vi "Solver1.vi"(10 "Word List":string[](array[string]), 11 "Word Search Grid":string[][](array[string])) -> (3 "Solutions":T2)   [LabVIEW 2022 SP3]
uses:
  support/Solutions--map.ctl
  support/Letter Index--cluster.ctl
panel:
  out "Array":T1[](array[typedef])
  # "Implement your Word Search challenge solution in this VI. Do not change the connector pane of this VI."
  # "Letters will always be ALL CAPS."
  # "Words will always be ALL CAPS."
  # "The Word Search Grid contains the 2D array of letters in which all words in the Word List appear. Words can appear forwards, backwards, up, down, and diagonally in any direction.\n\nThe Solutions map will contain one entry per item in the Word List. The map elements are:\n\nWord: The word from the Word List.\nLetter Indices: The row/column indices into the Word Search Grid for each letter (in order) in the word."
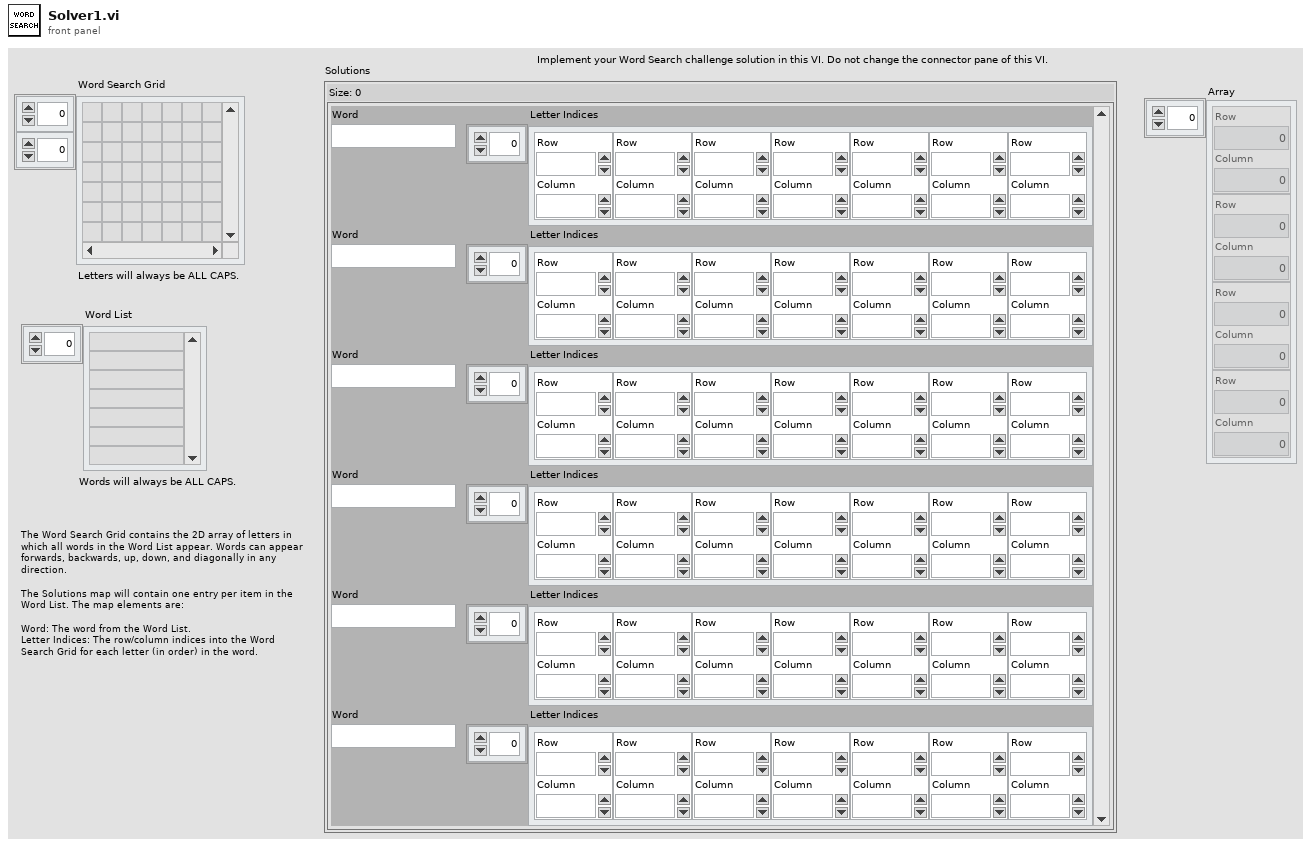
[diagram p1: front panel]
types:
  T1 = typedef "Letter Index--cluster.ctl" = cluster{"Row":i32, "Column":i32}
  T2 = typedef "Solutions--map.ctl" = map{string, T1[]}
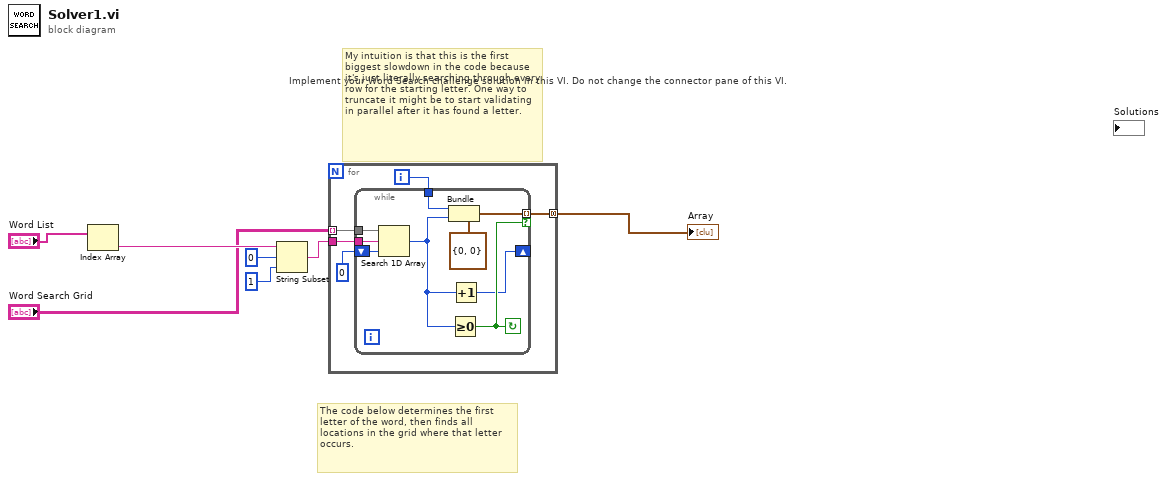
[diagram p0: block diagram]
diagram:
  # "My intuition is that this is the first biggest slowdown in the code because it's just literally searching through every row for the starting letter. One way to truncate it might be to start validating in parallel after it has found a letter."
  # "The code below determines the first letter of the word, then finds all locations in the grid where that letter occurs."
  # "Implement your Word Search challenge solution in this VI. Do not change the connector pane of this VI."
  n1 = Index Array(array="Word List") -> (element=w3:string)  [unwired: 1 in]
  n2 = String Subset(string=w3, offset (0)=0, length (rest)=1 ("length (rest)")) -> (substring=w6:string)
  n3 = for {
    tunnel: "Word Search Grid" -> [w12] mode=indexing
    tunnel: w6 -> [w11]
    tunnel: [w9] -> w1 mode=concatenating
    i -> [w10]
    n4 = while {
      tunnel: w12 -> [w21]
      tunnel: w11 -> [w20]
      tunnel: w10 -> [w18]
      tunnel: [w17] -> w9 mode=indexing if=w16
      shift-right: [w13] -> _
      shift-left: 0 -> [w15]
      stop <- w16 continue-if-true
      n5 = Search 1D Array(1D array=w21, element=w20, start index (0)=w15) -> (index of element=w14:i32)
      n6 = Bundle(cluster=T1 {"Row"=0, "Column"=0} ("Letter Index"), "Row"=w18, "Column"=w14) -> (w17:T1)
      n7 = Greater Or Equal To 0?(x=w14) -> (x >= 0?=w16:bool)
      n8 = Increment(x=w14) -> (x+1=w13:i32)
    }
  }
  "Array" <- w1
